vi "tearDown.vi"(8 "error in (no error)":errorcluster, 11 "reference in":refnum<class "Test-File IO.lvclass">) -> (0 "error out":errorcluster, 3 "reference out":refnum<class "Test-File IO.lvclass">)   [LabVIEW 2019, in "Test-File IO.lvclass"]
doc: "tearDown runs after the test method has completed. Use this method to clean up any operations or references that were opened by setUp or the test method. Unit tests should be independent of other unit tests so this VI should ensure that the next test can run in a 'clean' test environment."
uses:
  Test-File IO.lvclass
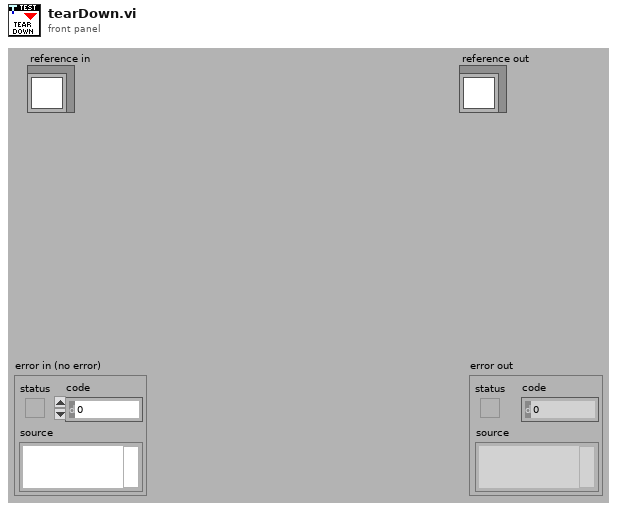
[diagram p1: front panel]
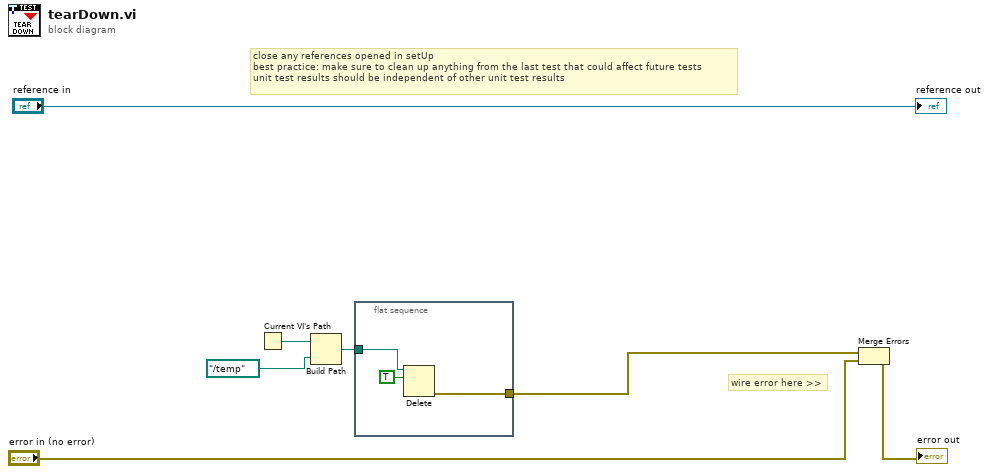
[diagram p0: block diagram]
diagram:
  # "wire error here >>"
  # "close any references opened in setUp\nbest practice: make sure to clean up anything from the last test that could affect future tests\nunit test results should be independent of other unit test results"
  n1 = Current VI's Path() -> (path=w3:path)
  n2 = Build Path(base path=w3, name or relative path=path "../temp") -> (appended path=w1:path)
  n3 = flat-sequence {
    tunnel: w1 -> [w10]
    tunnel: [w9] -> w4
    frame #0 {
      n4 = Delete(path (use dialog)=w10, entire hierarchy (F)=TRUE) -> (error out=w9:errorcluster)  [unwired: 3 in, 2 out]
    }
  }
  n5 = Merge Errors(w4, "error in (no error)") -> (→"error out":errorcluster)
  "reference out" <- "reference in"
